vi "Aero_WT_Temp_PID.vi"(1 "Change integral":bool, 2 "Present Value":dbl=15.0 format="%.2f", 3 "Previous Control Sum":dbl format="%.2f", 4 "Setpoint":dbl=15.0 format="%.2f") -> (0 "Dem Output":dbl format="%.2f")   [LabVIEW 2010]
uses:
  <vilib>/Analysis/NI_AALPro.lvlib
panel:
  in  "O/P deadband":dbl=1.0 format="%.2f"
  in  "Kp Deadband":dbl format="%.2f"
  in  "Derivative History":i32=120
  out "deadbanded error":dbl format="%.2f"
  in  "P":bool=TRUE
  in  "D":bool=TRUE
  in  "I":bool=TRUE
  out "Waveform Chart":T1(graph)
  in  "Manual Demand":dbl min=0.0 max=100.0 format="%.2f"
  in  "Manual Override":bool
  out "Control Sum":dbl format="%.2f"
  out "Derivative Term":dbl format="%.2f"
  out "Integral Term":dbl format="%.2f"
  out "error differential":dbl format="%.5f"
  out "error integral":dbl format="%.2f"
  out "Proportional Term":dbl format="%.2f"
  in  "Kd":dbl=300.0 format="%.2f"
  in  "Ki":dbl=3.0 format="%.2f"
  in  "Kp":dbl=10.0 format="%.2f"
  out "error":dbl format="%.2f"
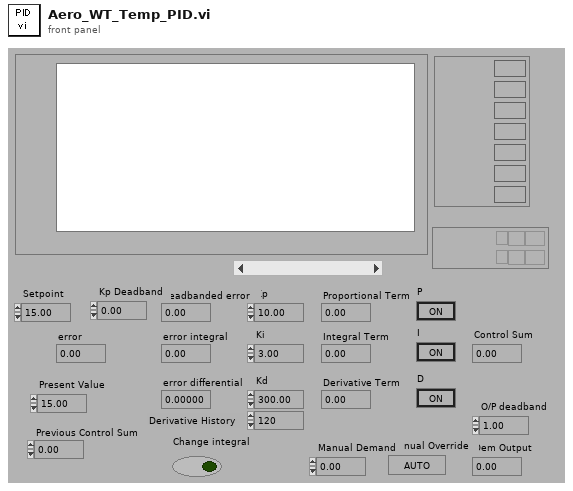
[diagram p1: front panel]
types:
  T1 = cluster{"Setpoint":dbl, "Present Value":dbl, "Proportional Term":dbl, "Integral Term":dbl, "Derivative Term":dbl, "Control Sum":dbl, "Dem Output":dbl}
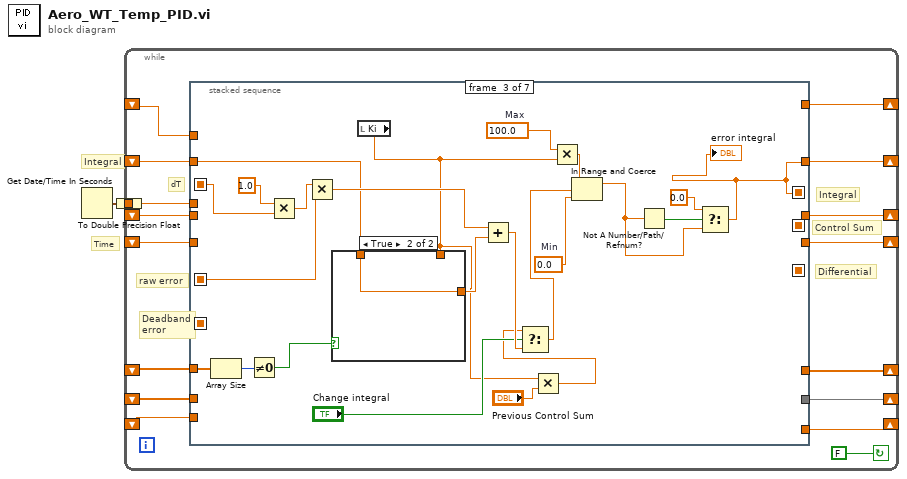
[diagram p0: block diagram]
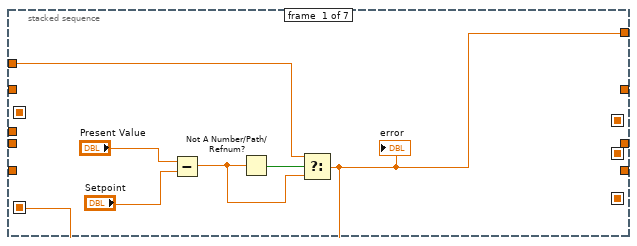
[diagram p2: hidden frame]
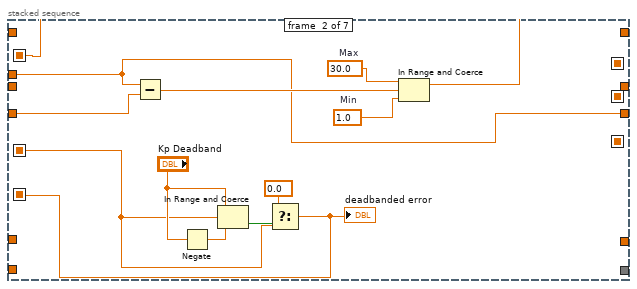
[diagram p3: hidden frame]
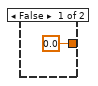
[diagram p4: hidden frame]
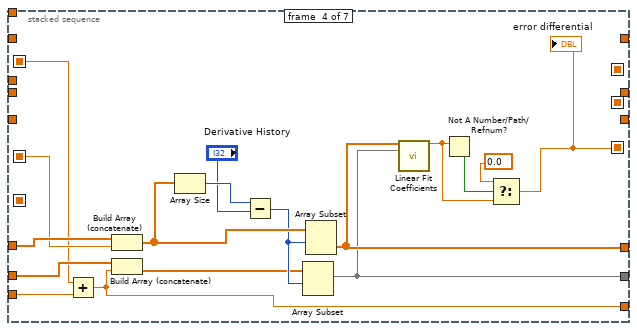
[diagram p5: hidden frame]
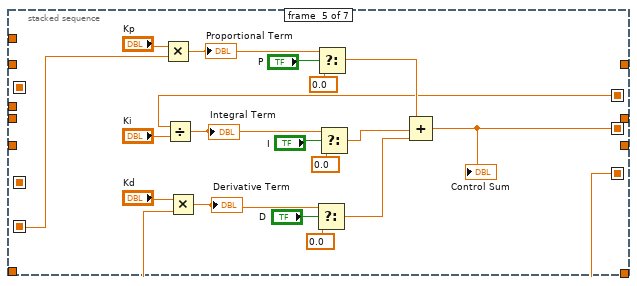
[diagram p6: hidden frame]
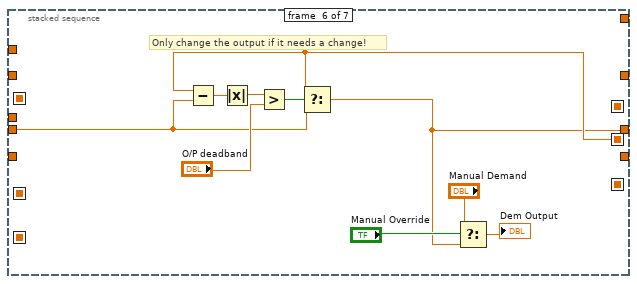
[diagram p7: hidden frame]
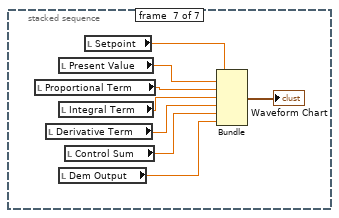
[diagram p8: hidden frame]
diagram:
  # "Integral"
  # "Time"
  n1 = Get Date/Time In Seconds() -> (seconds since 1Jan1904=w1:timestamp)
  n2 = To Double Precision Float(number=w1) -> (double precision float=w2:dbl)
  n3 = while {
    shift-left: _ -> [w5]
    shift-right: [w4] -> _
    shift-left: _ -> [w7]
    shift-right: [w6] -> _
    shift-left: _ -> [w9]
    shift-right: [w8] -> _
    tunnel: w2 -> [w14]
    shift-left: _ -> [w11]
    shift-right: [w10] -> _
    shift-left: _ -> [w13]
    shift-right: [w12] -> _
    shift-left: _ -> [w15]
    shift-right: [w16] -> _
    shift-left: _ -> [w18]
    shift-right: [w17] -> _
    stop <- FALSE continue-if-true
    # "Control Sum"
    # "raw error"
    # "Differential"
    # "Integral"
    # "Deadband\nerror"
    # "dT"
    n4 = stacked-sequence {
      seq-local: [_ w25 _ _ _ _ _] -> [_ _ w44 w64 _ _ _]
      seq-local: [_ w34 _ _ _ _ _] -> [_ _ _ _ w82 _ _]
      seq-local: [_ _ _ w69 _ _ _] -> [_ _ _ _ w81 _ _]
      seq-local: [_ _ w46 _ _ _ _] -> [_ _ _ _ w80 _ _]
      seq-local: [w19 _ _ _ _ _ _] -> [_ w26 w56 w70 _ _ _]
      seq-local: [_ _ _ _ w85 _ _] -> [_ _ _ _ _ w101 _]
      tunnel: w18 -> [_ w31 _ _ _ _ _]
      tunnel: [_ w29 _ _ _ _ _] -> w17
      tunnel: [_ _ w46 _ _ _ _] -> w16
      tunnel: w15 -> [_ _ w50 _ _ _ _]
      tunnel: w14 -> [_ w29 _ _ _ _ _]
      tunnel: w13 -> [_ _ w55 w78 _ _ _]
      tunnel: [_ _ _ w71 _ _ _] -> w12
      tunnel: w11 -> [_ _ _ w77 _ _ _]
      tunnel: [_ _ _ w68 _ _ _] -> w10
      tunnel: w9 -> [_ _ _ _ _ w99 _]
      tunnel: [_ _ _ _ _ w98 _] -> w8
      tunnel: w7 -> [_ _ _ w63 _ _ _]
      tunnel: [_ _ _ w62 _ _ _] -> w6
      tunnel: w5 -> [w21 _ _ _ _ _ _]
      tunnel: [w19 _ _ _ _ _ _] -> w4
      frame #0 {
        n5 = Subtract(x="Present Value", y="Setpoint") -> (x-y=w20:dbl)
        n6 = Not A Number/Path/Refnum?(number/path/refnum=w20) -> (NaN/Path/Refnum?=w22:bool)
        n7 = Select(t=w21, s=w22, f=w20) -> (s? t:f=w19:dbl)
        "error" <- w19
      }
      frame #1 {
        w32 = 1.0  # Min
        w33 = 30.0  # Max
        n8 = Subtract(x=w29, y=w31) -> (x-y=w30:dbl)
        n9 = Negate(x="Kp Deadband") -> (-x=w28:dbl)
        n10 = In Range and Coerce(upper limit="Kp Deadband", x=w26, lower limit=w28) -> (In Range?=w35:bool)  [unwired: 1 out]
        n11 = Select(t=0.0, s=w35, f=w26) -> (s? t:f=w34:dbl)
        "deadbanded error" <- w34
        n12 = In Range and Coerce(upper limit=w33, x=w30, lower limit=w32) -> (coerced(x)=w25:dbl)  [unwired: 1 out]
      }
      frame #2 {
        w59 = 0.0  # Min
        w58 = 100.0  # Max
        n13 = Array Size(array=w55) -> (size(s)=w54:i32)
        n14 = Not Equal To 0?(x=w54) -> (x != 0?=w52:bool)
        n15 = Multiply(x=1.0, y=w44) -> (x*y=w43:dbl)
        n16 = Multiply(x=w43, y=w56) -> (x*y=w53:dbl)
        n17 = local read "Ki"() -> (w38:dbl)
        n18 = case shown="True" w52 {
          tunnel: [0.0 ("Min") w61] -> w51
          tunnel: w50 -> [_ w61]
          tunnel: w38 -> [_ _]
          frame False {
          }
          frame True {
          }
        }
        n19 = Add(x=w53, y=w51) -> (x+y=w42:dbl)
        n20 = Multiply(x=w38, y="Previous Control Sum") -> (x*y=w37:dbl)
        n21 = Select(t=w37, s="Change integral", f=w42) -> (s? t:f=w40:dbl)
        n22 = Multiply(x=w58, y=w38) -> (x*y=w57:dbl)
        n23 = In Range and Coerce(upper limit=w57, x=w40, lower limit=w59) -> (coerced(x)=w47:dbl)  [unwired: 1 out]
        n24 = Not A Number/Path/Refnum?(number/path/refnum=w47) -> (NaN/Path/Refnum?=w48:bool)
        n25 = Select(t=0.0, s=w48, f=w47) -> (s? t:f=w46:dbl)
        "error integral" <- w46
      }
      frame #3 {
        n26 = Add(x=w64, y=w63) -> (x+y=w62:dbl)
        n27 = Build Array (concatenate)(w78, w70) -> (w74:dbl[])
        n28 = Build Array (concatenate)(w77, w62) -> (w72:dbl[])
        n29 = Array Size(array=w74) -> (size(s)=w76:i32)
        n30 = Subtract(x=w76, y="Derivative History") -> (x-y=w73:i32)
        n31 = Array Subset(array=w72, index=w73) -> (w68:dbl[])  [unwired: 1 in]
        n32 = Array Subset(array=w74, index=w73) -> (w71:dbl[])  [unwired: 1 in]
        n33 = call <vilib>:"Linear Fit Coefficients.vi"("Y"=w71, "X"=w68) -> ("slope"=w65:dbl)  [unwired: 3 in, 10 out]
        n34 = Not A Number/Path/Refnum?(number/path/refnum=w65) -> (NaN/Path/Refnum?=w67:bool)
        n35 = Select(t=0.0 ("f"), s=w67, f=w65) -> (s? t:f=w69:dbl)
        "error differential" <- w69
      }
      frame #4 {
        n36 = Multiply(x="Kp", y=w82) -> (x*y=w95:dbl)
        "Proportional Term" <- w95
        n37 = Divide(x=w80, y="Ki") -> (x/y=w86:dbl)
        "Integral Term" <- w86
        n38 = Multiply(x="Kd", y=w81) -> (x*y=w87:dbl)
        "Derivative Term" <- w87
        n39 = Select(t=w87, s="D", f=0.0) -> (s? t:f=w89:dbl)
        n40 = Select(t=w95, s="P", f=0.0) -> (s? t:f=w96:dbl)
        n41 = Select(t=w86, s="I", f=0.0) -> (s? t:f=w88:dbl)
        n42 = Compound Arithmetic op=ADD(w96, w88, w89) -> (w85:dbl)
        "Control Sum" <- w85
      }
      frame #5 {
        # "Only change the output if it needs a change!"
        n43 = Subtract(x=w101, y=w99) -> (x-y=w104:dbl)
        n44 = Absolute Value(x=w104) -> (abs(x)=w103:dbl)
        n45 = Greater?(x=w103, y="O/P deadband") -> (0:w102:bool)
        n46 = Select(t=w101, s=w102, f=w99) -> (s? t:f=w98:dbl)
        n47 = Select(t="Manual Demand", s="Manual Override", f=w98) -> (s? t:f=→"Dem Output":dbl)
      }
      frame #6 {
        n48 = local read "Proportional Term"() -> (w111:dbl)
        n49 = local read "Derivative Term"() -> (w113:dbl)
        n50 = local read "Present Value"() -> (w110:dbl)
        n51 = local read "Integral Term"() -> (w112:dbl)
        n52 = local read "Dem Output"() -> (w115:dbl)
        n53 = local read "Control Sum"() -> (w114:dbl)
        n54 = local read "Setpoint"() -> (w109:dbl)
        n55 = Bundle("Setpoint"=w109, "Present Value"=w110, "Proportional Term"=w111, "Integral Term"=w112, "Derivative Term"=w113, "Control Sum"=w114, "Dem Output"=w115) -> (→"Waveform Chart":T1)  [unwired: 1 out]
      }
    }
  }
